vi "Write setting file.vi"(8 "error in (no error)":errorcluster, 9 "Ackstatus":i32, 10 "Action":i32, 11 "Setring file path":path) -> (0 "error out":errorcluster)   [LabVIEW 2012]
panel:
  out "子字符串之前":string
  out "result string 2":string
  out "text":string
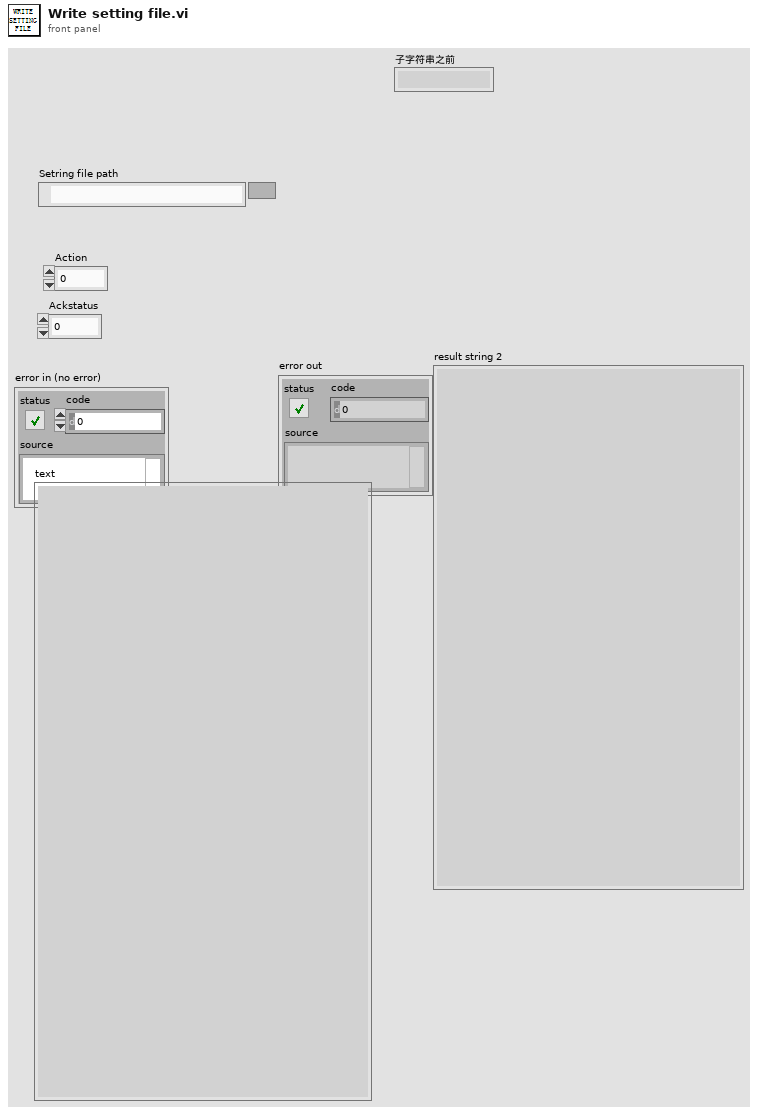
[diagram p1: front panel]
types:
  T1 = enum16{"open", "replace", "create", "open or create", "replace or create", "replace or create with confirmation"}
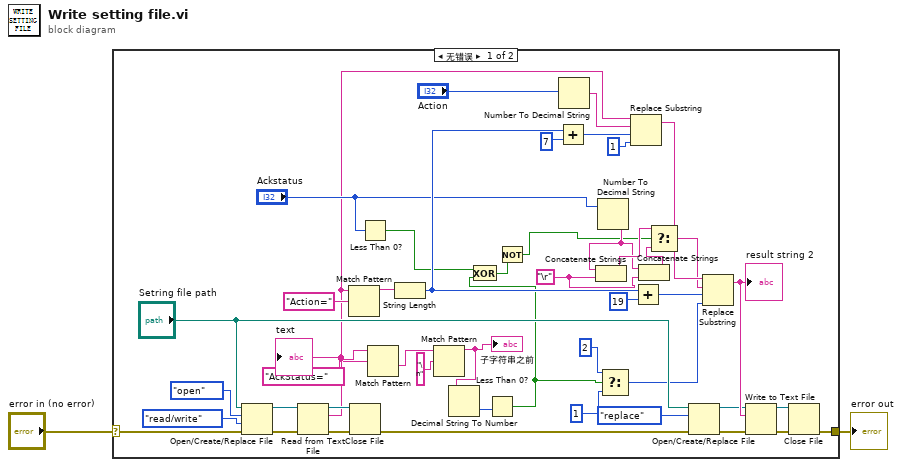
[diagram p0: block diagram]
diagram:
  n1 = case shown="无错误" "error in (no error)" {
    selector: "error in (no error)" -> [w44 _]
    tunnel: [w24 _] -> w1
    frame No Error {
      w14 = "\r"
      n2 = Open/Create/Replace File(file path (use dialog)="Setring file path", error in=w44, operation (0:open)=T1."open", access (0:read/write)=enum16{"read/write", "read-only", "write-only"}."read/write") -> (refnum out=w46:refnum<file>, error out=w45:errorcluster)  [unwired: 2 in, 1 out]
      n3 = Read from Text File(file (use dialog)=w46, error in=w45) -> (refnum out=w33:refnum<file>, text=w12:string, error out=w32:errorcluster)  [unwired: 2 in, 1 out]
      "text" <- w12
      n4 = Match Pattern(string=w12, regular expression="Action=") -> (before substring=w43:string)  [unwired: 1 in, 3 out]
      n5 = Close File(refnum=w33, error in=w32) -> (error out=w28:errorcluster)  [unwired: 1 out]
      n6 = Less Than 0?(x="Ackstatus") -> (x < 0?=w6:bool)
      n7 = Match Pattern(string=w12, regular expression="AckStatus=" ("正则表达式")) -> (after substring=w10:string)  [unwired: 1 in, 3 out]
      n8 = String Length(string=w43) -> (length=w38:i32)
      n9 = Match Pattern(string=w10, regular expression="\n" ("正则表达式")) -> (before substring=w7:string)  [unwired: 1 in, 3 out]
      "子字符串之前" <- w7
      n10 = Decimal String To Number(string=w7) -> (number=w8:i32)  [unwired: 2 in, 1 out]
      n11 = Less Than 0?(x=w8) -> (x < 0?=w3:bool)
      n12 = Exclusive Or(1:w3, 2:w6) -> (0:w5:bool)
      n13 = Not(x=w5) -> (.not. x?=w4:bool)
      n14 = Add(x=w38, y=7) -> (x+y=w39:i32)
      n15 = Number To Decimal String(number="Action") -> (decimal integer string=w41:string)  [unwired: 1 in]
      n16 = Number To Decimal String(number="Ackstatus") -> (decimal integer string=w15:string)  [unwired: 1 in]
      n17 = Concatenate Strings(w15, w14) -> (w18:string)
      n18 = Select(t=2 ("length (len. of substring)"), s=w3, f=1) -> (s? t:f=w20:i32)
      n19 = Replace Substring(2:1 ("length (len. of substring)"), 3:w39, 4:w41, 5:w12) -> (1:w35:string)  [unwired: 1 out]
      n20 = Add(x=w38, y=19) -> (x+y=w19:i32)
      n21 = Concatenate Strings(w15, w14) -> (w16:string)
      n22 = Select(t=w18, s=w4, f=w16) -> (s? t:f=w17:string)
      n23 = Open/Create/Replace File(file path (use dialog)="Setring file path", error in=w28, operation (0:open)=T1."replace") -> (refnum out=w29:refnum<file>, error out=w27:errorcluster)  [unwired: 3 in, 1 out]
      n24 = Replace Substring(2:w20, 3:w19, 4:w17, 5:w35) -> (1:w34:string)  [unwired: 1 out]
      "result string 2" <- w34
      n25 = Write to Text File(file (use dialog)=w29, text=w34, error in=w27) -> (refnum out=w25:refnum<file>, error out=w26:errorcluster)  [unwired: 1 in, 1 out]
      n26 = Close File(refnum=w25, error in=w26) -> (error out=w24:errorcluster)  [unwired: 1 out]
    }
    frame Error {
    }
  }
  "error out" <- w1
